vi "HTML_GetFramework_CSS_JS_Dependencies.vi"(7 "Framwork Type":T1) -> (1 "rel. Filepaths .js":path[](array[path]), 2 "rel. Filepaths .css":path[](array[path]))   [LabVIEW 2014]
uses:
  controls/StylingFrameworks_Enum.ctl
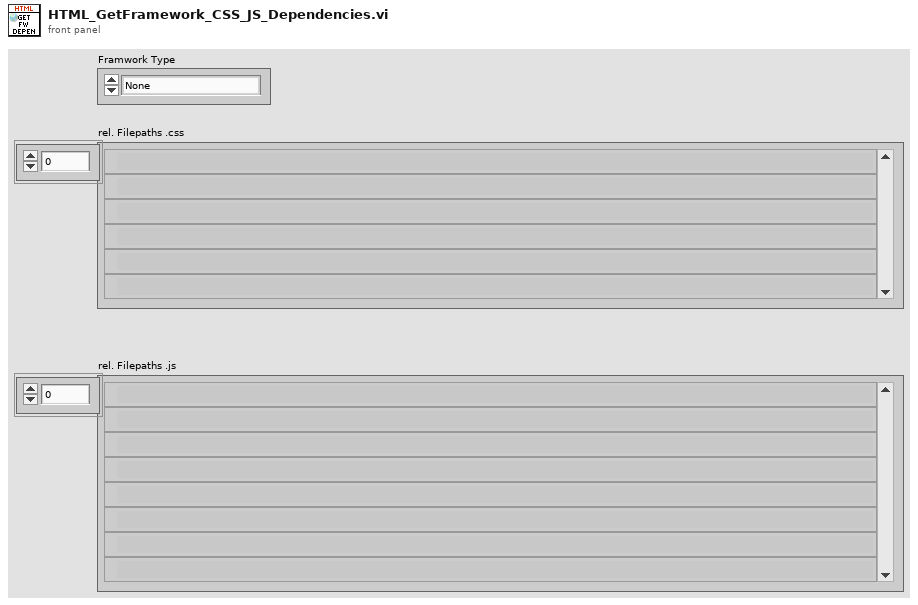
[diagram p1: front panel]
types:
  T1 = typedef "StylingFrameworks_Enum.ctl" = enum16{"None", "Bootstrap4", "Semantic-UI", "Custom"}
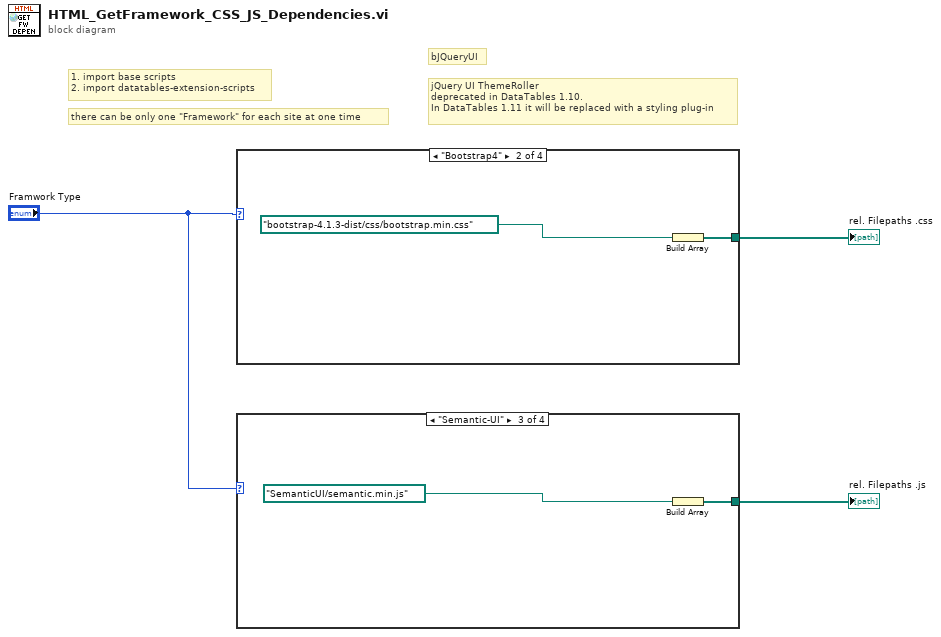
[diagram p0: block diagram]
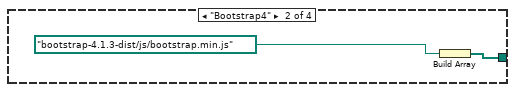
[diagram p3: hidden frame]
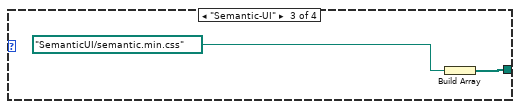
[diagram p6: hidden frame]
diagram:
  # "jQuery UI ThemeRoller\ndeprecated in DataTables 1.10. \nIn DataTables 1.11 it will be replaced with a styling plug-in"
  # "bJQueryUI"
  # "there can be only one \"Framework\" for each site at one time"
  # "1. import base scripts\n2. import datatables-extension-scripts"
  n1 = case shown="\"Bootstrap4\"" "Framwork Type" {
    tunnel: [_ w4 w6 _] -> w3
    frame "None", Default {
    }
    frame "Bootstrap4" {
      n2 = Build Array(path "bootstrap-4.1.3-dist/css/bootstrap.min.css") -> (w4:path[])
    }
    frame "Semantic-UI" {
      n3 = Build Array(path "SemanticUI/semantic.min.css") -> (w6:path[])
    }
    frame "Custom" {
    }
  }
  "rel. Filepaths .css" <- w3
  n4 = case shown="\"Semantic-UI\"" "Framwork Type" {
    tunnel: [_ w8 w10 _] -> w1
    frame "None", Default {
    }
    frame "Bootstrap4" {
      n5 = Build Array(path "bootstrap-4.1.3-dist/js/bootstrap.min.js") -> (w8:path[])
    }
    frame "Semantic-UI" {
      n6 = Build Array(path "SemanticUI/semantic.min.js") -> (w10:path[])
    }
    frame "Custom" {
    }
  }
  "rel. Filepaths .js" <- w1
